vi "PeriodicFilter-Update Filtered Info.vi"(11 "data in":T1 {"LastCheckT" format="%<%.3X>T"}) -> (3 "data out":T1 {"LastCheckT" format="%<%.3X>T"})   [LabVIEW 2017, in "Communicable State Machine.lvlib"]
uses:
  Communicable State Machine.lvlib
  Periodic String Filter Data.ctl
  Periodic String Filter Info.ctl
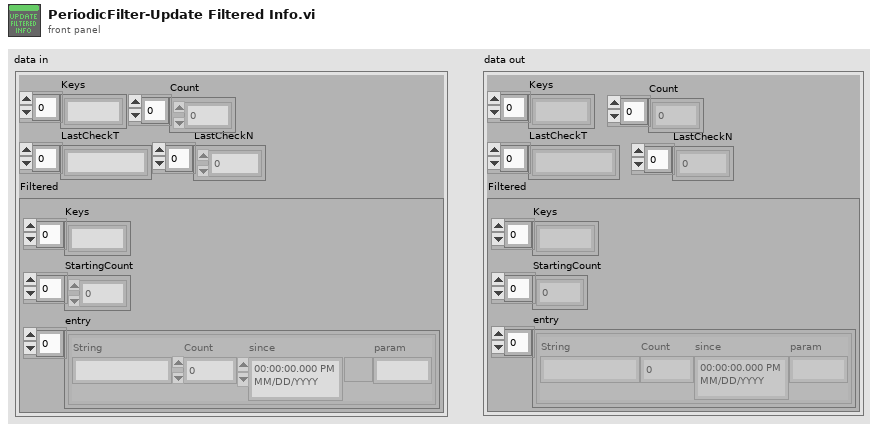
[diagram p1: front panel]
types:
  T1 = typedef "Communicable State Machine.lvlib/Periodic String Filter Data.ctl" = cluster{"Keys":string[], "Count":i64[], "LastCheckT":timestamp[], "LastCheckN":i64[], "Filtered":cluster{"Keys":string[], "StartingCount":i64[], "entry":T2[]}}
  T2 = typedef "Communicable State Machine.lvlib/Periodic String Filter Info.ctl" = cluster{"String":string, "Count":i64, "since":timestamp, "param":string}
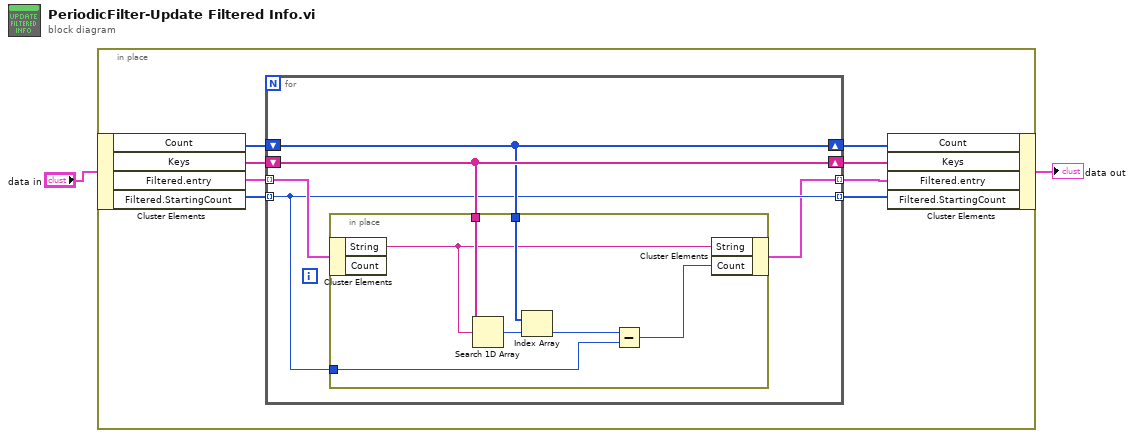
[diagram p0: block diagram]
diagram:
  n1 = in-place "In Place Element Structure" {
    n2 = in-place-cluster #1("data in") -> ("Count"=w8:i64[], "Keys"=w10:string[], "Filtered.entry"=w6:T2[], "Filtered.StartingCount"=w5:i64[])
    n3 = for {
      shift-right: [w15] -> w9
      shift-left: w10 -> [w15]
      shift-right: [w14] -> w7
      shift-left: w8 -> [w14]
      tunnel: w6 -> [w13] mode=indexing
      tunnel: w5 -> [w12] mode=indexing
      tunnel: [w12] -> w4 mode=indexing
      tunnel: [w11] -> w3 mode=indexing
      n4 = in-place {
        in-place-border: w12 -> [w20]
        in-place-border: w15 -> [w19]
        in-place-border: w14 -> [w18]
        n5 = in-place-cluster #2(w13) -> ("String"=w16:string)  [unwired: 1 out]
        n6 = Search 1D Array(1D array=w19, element=w16) -> (index of element=w22:i32)  [unwired: 1 in]
        n7 = Index Array(array=w18, index=w22) -> (element=w21:i64)
        n8 = Subtract(x=w21, y=w20) -> (x-y=w17:i64)
        n9 = in-place-cluster #2("String"=w16, "Count"=w17) -> (w11:T2)
      }
    }
    n10 = in-place-cluster #1("Count"=w7, "Keys"=w9, "Filtered.entry"=w3, "Filtered.StartingCount"=w4) -> (→"data out":T1)
  }
